vi "split sql statements.vi"(10 "Multiple SQL statements in":string) -> (1 "#statements":i32, 2 "Individual SQL statements out":string[](array[string]))   [LabVIEW 2020, in "sqlite3.lvlib"]
uses:
  sqlite3/Source/sqlite3.lvlib
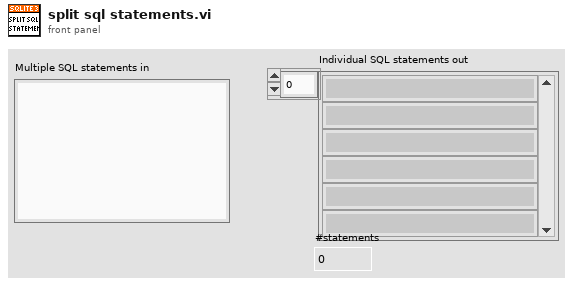
[diagram p1: front panel]
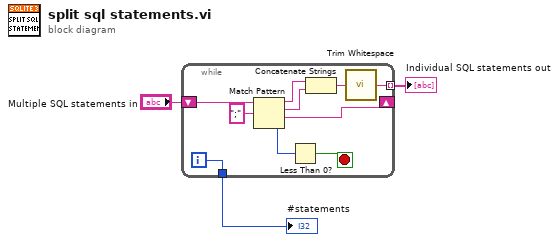
[diagram p0: block diagram]
diagram:
  n1 = while {
    shift-right: [w9] -> _
    shift-left: "Multiple SQL statements in" -> [w13]
    tunnel: [w5] -> w2 mode=indexing
    tunnel: [w4] -> w1
    i -> [w4]
    stop <- w10 stop-if-true
    n2 = Match Pattern(string=w13, regular expression=";") -> (before substring=w8:string, match substring=w7:string, after substring=w9:string, offset past match=w11:i32)  [unwired: 1 in]
    n3 = Less Than 0?(x=w11) -> (x < 0?=w10:bool)
    n4 = Concatenate Strings(w8, w7) -> (w6:string)
    n5 = call <vilib>:"Trim Whitespace.vi"("string"=w6) -> ("trimmed string"=w5:string)  [unwired: 1 in]
  }
  "Individual SQL statements out" <- w2
  "#statements" <- w1
